vi "Combined Algorithm.vi"() -> ()   [LabVIEW 2020]
uses:
  <vilib>/MakerHub/LINX/Private/Type Defs/Peripherals/SPI/SPI Configuration.ctl
  <vilib>/MakerHub/LINX/Private/Type Defs/Peripherals/SPI/SPI Bit Order.ctl
  <vilib>/MakerHub/LINX/Private/Type Defs/Peripherals/SPI/SPI Mode.ctl
  <vilib>/MakerHub/LINX/Public/Peripherals/SPI/SPI CS Config.ctl
  <vilib>/MakerHub/LINX/Private/Type Defs/Peripherals/SPI/SPI CS Logic Level.ctl
  <vilib>/MakerHub/LINX/Public/Peripherals/Analog/Analog Read 1 Chan.vi
  <vilib>/MakerHub/LINX/Public/Peripherals/SPI/SPI Write Read 1 Frame.vi
  <vilib>/MakerHub/LINX/Public/Peripherals/PWM/PWM Set Duty Cycle 1 Chan.vi
  <vilib>/MakerHub/LINX/Public/Peripherals/Digital/Digital Write 1 Chan.vi
  <vilib>/MakerHub/LINX/Public/Peripherals/Analog/Analog Read N Chans.vi
  <vilib>/MakerHub/LINX/Public/Peripherals/SPI/SPI Write Read N Frames.vi
  <vilib>/MakerHub/LINX/Public/Peripherals/Digital/Digital Write N Chans.vi
  <vilib>/MakerHub/LINX/Private/Local IO/LinxAnalogRead.vi
  <vilib>/MakerHub/LINX/Public/Utilities/Check Channel.vi
  <vilib>/MakerHub/LINX/Private/Local IO/LinxSpiWriteRead.vi
  <vilib>/MakerHub/LINX/Private/Local IO/LinxDigitalWrite.vi
  <vilib>/MakerHub/LINX/Public/Utilities/Open Serial.vi
  <vilib>/MakerHub/LINX/Private/Utilties/Generate Error.vi
  <vilib>/MakerHub/LINX/Public/Peripherals/PWM/PWM Set Duty Cycle N Chans.vi
  <vilib>/MakerHub/LINX/LMH-LINX.lvlib
panel:
  in  "DO Channel -  Exhaust Fan":u8
  in  "DO Channel - Solar Water Motor":u8
  in  "IR sensor Analog Channel (A0)":u8
  out "IR Sensor (Fire detected)":bool
  out "IR Sensor output voltage":dbl
  in  "PWM Channel - Buzzer":u8
  in  "Smoke Threshold":dbl
  out "Smoke sensor output Voltage":dbl
  in  "Smoke sensor Analog Channel(A2)":u8
  out "Temperature":dbl
  in  "stop":bool
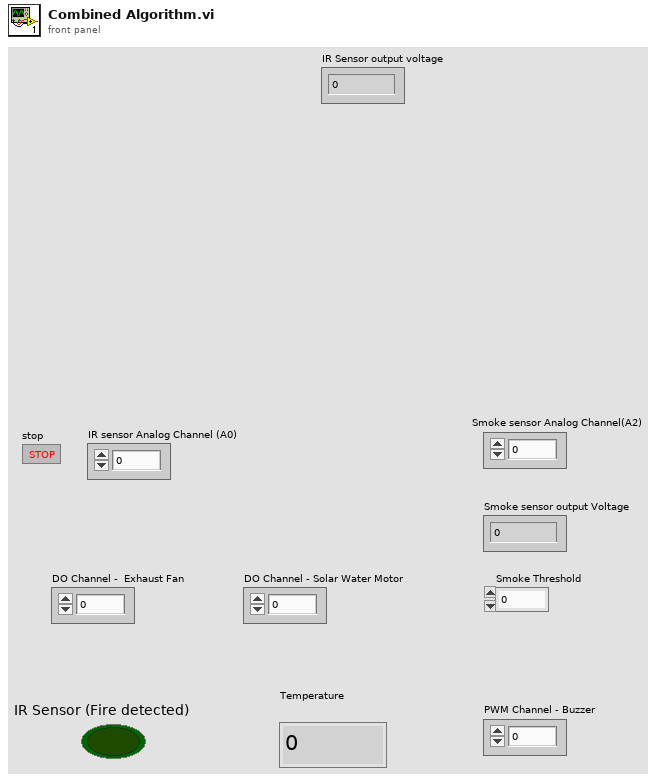
[diagram p1: front panel]
types:
  T1 = typedef "LMH-LINX.lvlib/SPI Configuration.ctl" = cluster{"Clock Frequency":u32, "Bit Order":T2, "SPI Mode":T3}
  T2 = typedef "LMH-LINX.lvlib/SPI Bit Order.ctl" = enum8{"LSb First", "MSb First"}
  T3 = typedef "LMH-LINX.lvlib/SPI Mode.ctl" = enum8{"Mode 0", "Mode 1", "Mode 2", "Mode 3"}
  T4 = typedef "LMH-LINX.lvlib/LINX Ref.ctl" = cluster{"IO":T5, "Interface":T6, "LINX Device Config":T7}
  T5 = typedef "LMH-LINX.lvlib/Platform.ctl" = enum16{"Remote", "Local"}
  T6 = typedef "LMH-LINX.lvlib/Interface.ctl" = enum16{"Serial", "TCP"}
  T7 = typedef "LMH-LINX.lvlib/Device.lvlib/LINX Device Config.ctl" = cluster{"Interface":T6, "COM Port":refnum<visa-resource-name>, "TCP Configuration":T8, "Device Family":u8, "Device ID":u8, "Device Name":string, "TCP Ref":refnum<k5>, "Channels":T9}
  T8 = typedef "LMH-LINX.lvlib/Device.lvlib/TCP Config.ctl" = cluster{"IP Address":string, "Port":u16}
  T9 = typedef "LMH-LINX.lvlib/Channels.ctl" = cluster{"DI":u8[], "DO":u8[], "AI":u8[], "AO":u8[], "PWM":u8[], "QE":u8[], "UART":u8[], "I2C 2":u8[], "SPI":u8[], "CAN":u8[], "Servo":u8[], "AI Ref (V)":dbl, "AI Resolution (Bits)":u8, "AO Ref (V)":dbl, "AO Resolution (Bits)":u8}
  T10 = typedef "LMH-LINX.lvlib/SPI CS Config.ctl" = cluster{"CS Channel":u8, "CS Logic Level":T11}
  T11 = typedef "LMH-LINX.lvlib/SPI CS Logic Level.ctl" = enum8{"Active Low", "Active High"}
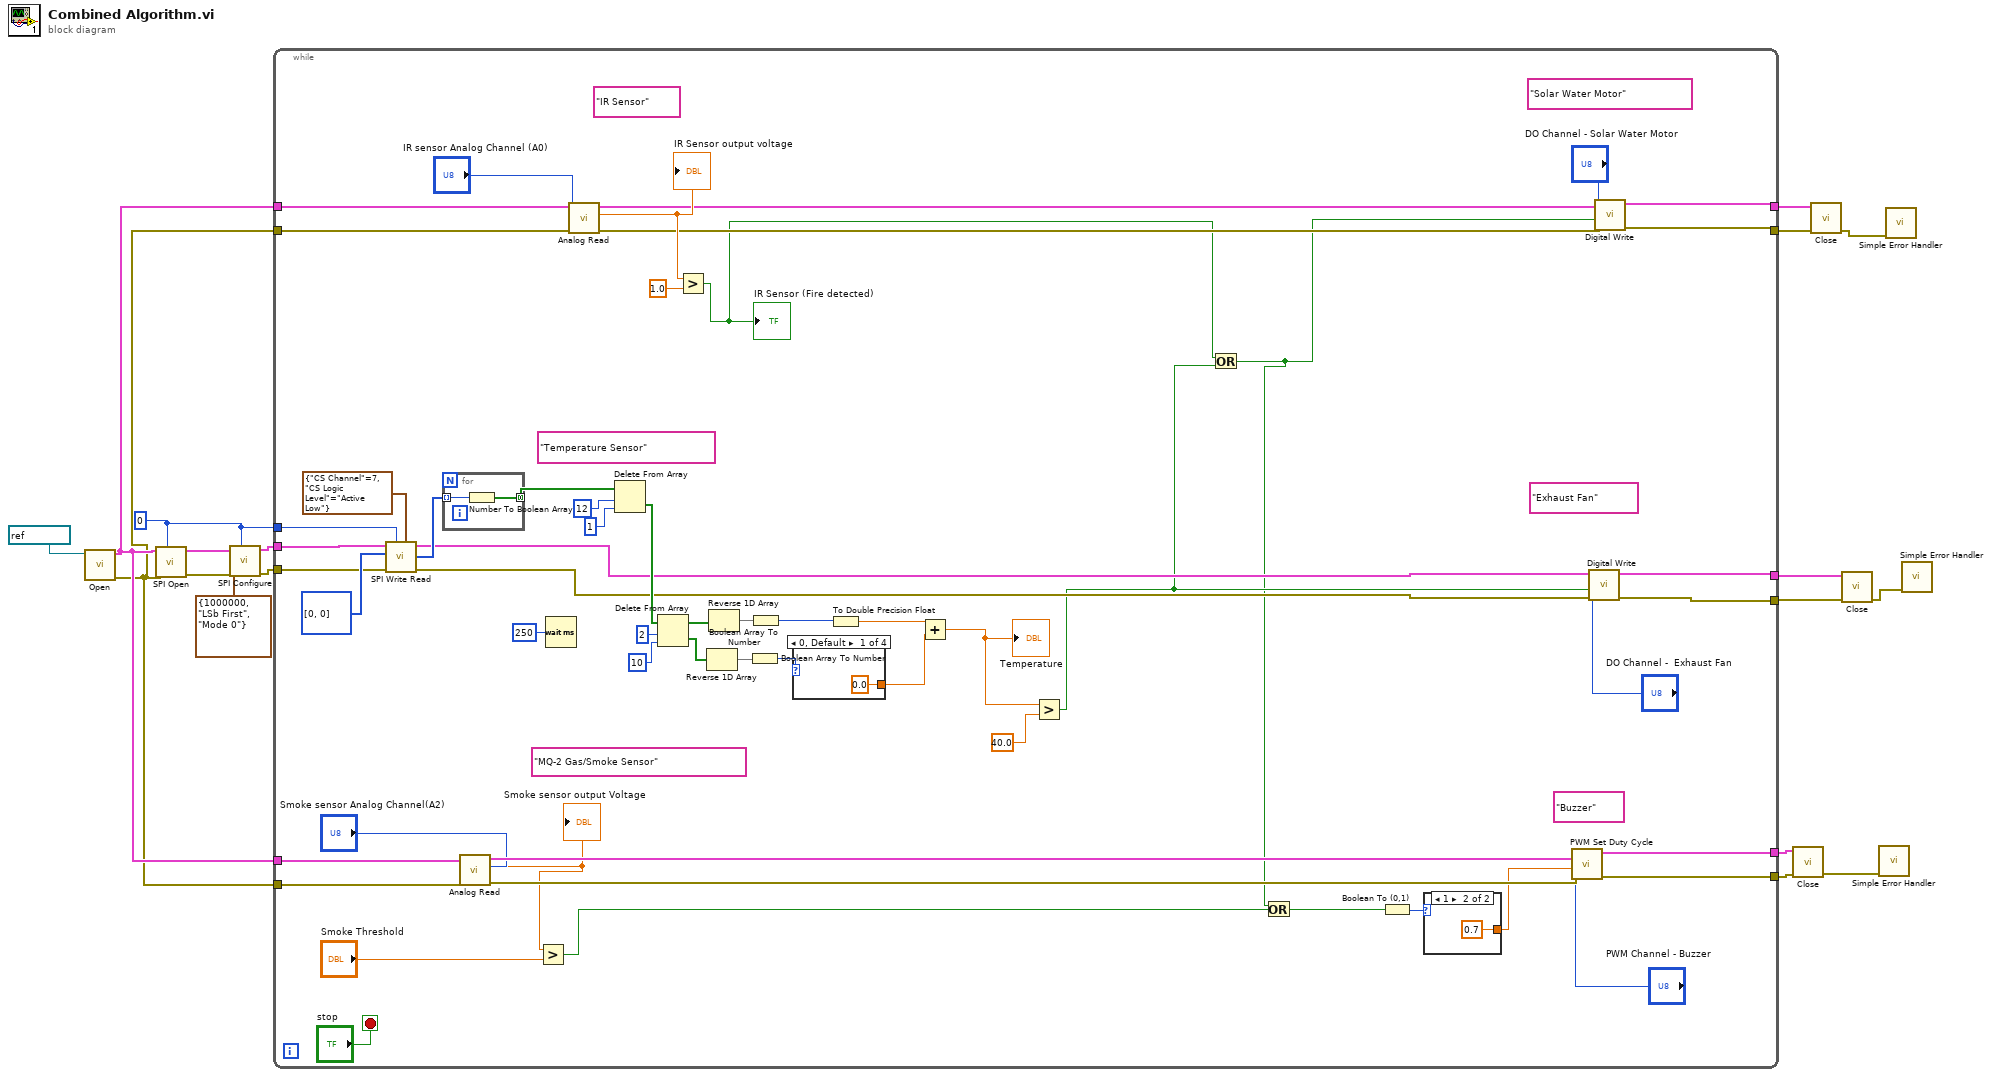
[diagram p0: block diagram]
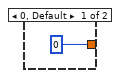
[diagram p2: hidden frame]
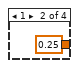
[diagram p3: hidden frame]
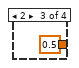
[diagram p4: hidden frame]
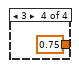
[diagram p5: hidden frame]
diagram:
  w12 = u8 0 ("SPI Channel (0)")
  n1 = call-poly <vilib>:"Open.vi"("Serial Port"=refnum<visa-resource-name> "COM3") -> ("Error Out"=w7:errorcluster, "LINX Resource"=w8:T4)  [unwired: 8 in, 1 out]
  n2 = call <vilib>:"SPI Open.vi"("SPI Channel (0)"=w12, "Error In"=w7, "LINX Resource"=w8) -> ("Error Out"=w17:errorcluster, "LINX Resource"=w16:T4)  [unwired: 7 in]
  n3 = call <vilib>:"SPI Configure.vi"("SPI Channel (0)"=w12, "Error In"=w17, "SPI Configuration"=T1 {"Clock Frequency"=1000000, "Bit Order"=enum."LSb First", "SPI Mode"=enum."Mode 0"}, "LINX Resource"=w16) -> ("Error Out"=w14:errorcluster, "LINX Resource"=w15:T4)  [unwired: 5 in, 1 out]
  n4 = while {
    tunnel: w15 -> [w73]
    tunnel: [w29] -> w4
    tunnel: w14 -> [w55]
    tunnel: [w28] -> w13
    tunnel: w12 -> [w54]
    tunnel: w8 -> [w46]
    tunnel: w7 -> [w45]
    tunnel: [w43] -> w10
    tunnel: [w42] -> w9
    tunnel: w8 -> [w39]
    tunnel: w7 -> [w38]
    tunnel: [w34] -> w6
    tunnel: [w33] -> w5
    stop <- "stop" stop-if-true
    (unwired) "Exhaust Fan"
    (unwired) "Buzzer"
    (unwired) "Solar Water Motor"
    (unwired) "IR Sensor"
    (unwired) "Temperature Sensor"
    (unwired) "MQ-2 Gas/Smoke Sensor"
    n5 = call-poly <vilib>:"SPI Write Read.vi"("CS Configuration"=T10 {"CS Channel"=7, "CS Logic Level"=enum."Active Low"}, "SPI Channel (0)"=w54, "Error In"=w55, "Data"=u16[] [0, 0], "LINX Resource"=w73) -> ("Error Out"=w30:errorcluster, "Read Data"=w71:u8[], "LINX Resource"=w31:T4)  [unwired: 4 in]
    n6 = for {
      tunnel: w71 -> [w82] mode=indexing
      tunnel: [w81] -> w53 mode=concatenating
      n7 = Number To Boolean Array(number=w82) -> (Boolean array=w81:bool[])
    }
    n8 = call-poly <vilib>:"Analog Read.vi"("Error In"=w45, "Analog Channel"="Smoke sensor Analog Channel(A2)", "LINX Resource"=w46) -> ("Error Out"=w51:errorcluster, "Voltage"=w49:dbl, "LINX Resource"=w52:T4)  [unwired: 5 in, 1 out]
    "Smoke sensor output Voltage" <- w49
    n9 = Greater?(x=w49, y="Smoke Threshold") -> (0:w21:bool)
    n10 = Wait (ms)(milliseconds to wait=u32 250) -> ()  [unwired: 1 out]
    n11 = call-poly <vilib>:"Analog Read.vi"("Error In"=w38, "Analog Channel"="IR sensor Analog Channel (A0)", "LINX Resource"=w39) -> ("Error Out"=w35:errorcluster, "Voltage"=w41:dbl, "LINX Resource"=w36:T4)  [unwired: 5 in, 1 out]
    "IR Sensor output voltage" <- w41
    n12 = Delete From Array(array=w53, length=12, index=1) -> (deleted portion=w66:bool[])  [unwired: 1 out]
    n13 = Delete From Array(array=w66, length=2, index=10) -> (deleted portion=w62:bool[], array with subset deleted=w63:bool[])
    n14 = Greater?(x=w41, y=1.0) -> (0:w24:bool)
    "IR Sensor (Fire detected)" <- w24
    n15 = Reverse 1D Array(array=w62) -> (reversed array=w60:bool[])
    n16 = Reverse 1D Array(array=w63) -> (reversed array=w61:bool[])
    n17 = Boolean Array To Number(Boolean array=w60) -> (number=w59:u32)
    n18 = Boolean Array To Number(Boolean array=w61) -> (number=w56:u32)
    n19 = case shown="0, Default" w59 {
      tunnel: [0.0 0.25 0.5 0.75] -> w58
      frame 0, Default {
      }
      frame 1 {
      }
      frame 2 {
      }
      frame 3 {
      }
    }
    n20 = To Double Precision Float(number=w56) -> (double precision float=w57:dbl)
    n21 = Add(x=w57, y=w58) -> (x+y=w27:dbl)
    "Temperature" <- w27
    n22 = Greater?(x=w27, y=40.0) -> (0:w23:bool)
    n23 = Or(x=w24, y=w23) -> (x .or. y?=w19:bool)
    n24 = Or(x=w19, y=w21) -> (x .or. y?=w20:bool)
    n25 = Boolean To (0,1)(Boolean=w20) -> (0, 1=w48:i16)
    n26 = case shown="1" w48 {
      tunnel: [0 0.7] -> w22
      frame 0, Default {
      }
      frame 1 {
      }
    }
    n27 = call-poly <vilib>:"PWM Set Duty Cycle.vi"("Error In"=w51, "Duty Cycle (0-1)"=w22, "PWM Channel"="PWM Channel - Buzzer", "LINX Resource"=w52) -> ("Error Out"=w42:errorcluster, "LINX Resource"=w43:T4)  [unwired: 6 in]
    n28 = call-poly <vilib>:"Digital Write.vi"("Error In"=w30, "Output Value"=w23, "DO Channel"="DO Channel -  Exhaust Fan", "LINX Resource"=w31) -> ("Error Out"=w28:errorcluster, "LINX Resource"=w29:T4)  [unwired: 6 in]
    n29 = call-poly <vilib>:"Digital Write.vi"("Error In"=w35, "Output Value"=w19, "DO Channel"="DO Channel - Solar Water Motor", "LINX Resource"=w36) -> ("Error Out"=w33:errorcluster, "LINX Resource"=w34:T4)  [unwired: 6 in]
  }
  n30 = call <vilib>:"Close.vi"("Error In"=w9, "LINX Resource"=w10) -> ("Error Out"=w3:errorcluster)  [unwired: 9 in]
  n31 = call <vilib>:"Close.vi"("Error In"=w5, "LINX Resource"=w6) -> ("Error Out"=w1:errorcluster)  [unwired: 9 in]
  n32 = call <vilib>:"Close.vi"("Error In"=w13, "LINX Resource"=w4) -> ("Error Out"=w2:errorcluster)  [unwired: 9 in]
  n33 = call <vilib>:"Simple Error Handler.vi"("error in (no error)"=w3) -> ()  [unwired: 4 in, 5 out]
  n34 = call <vilib>:"Simple Error Handler.vi"("error in (no error)"=w1) -> ()  [unwired: 4 in, 5 out]
  n35 = call <vilib>:"Simple Error Handler.vi"("error in (no error)"=w2) -> ()  [unwired: 4 in, 5 out]
